vi "Calc - DPPbvi.vi"(10 "PBMeas P":dbl format="%#_13g", 11 "PBAR":dbl format="%#_13g") -> (3 "DPPb":dbl)   [LabVIEW 2018, in "Controller (Host).lvlib"]
uses:
  Controller (Host).lvlib
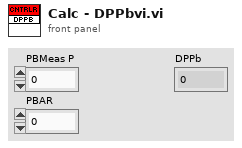
[diagram p1: front panel]
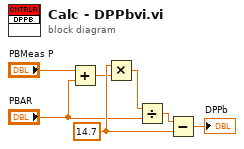
[diagram p0: block diagram]
diagram:
  w7 = 14.7 ("x")
  n1 = Add(x="PBMeas P", y="PBAR") -> (x+y=w4:dbl)
  n2 = Multiply(x=w7, y=w4) -> (x*y=w5:dbl)
  n3 = Divide(x=w5, y="PBAR") -> (x/y=w6:dbl)
  n4 = Subtract(x=w6, y=w7) -> (x-y=→"DPPb":dbl)
